vi "test.vi"() -> ()   [LabVIEW 2020]
panel:
  out "Array":i32[][](array[numeric])
  out "transposed array":i32[][](array[numeric])
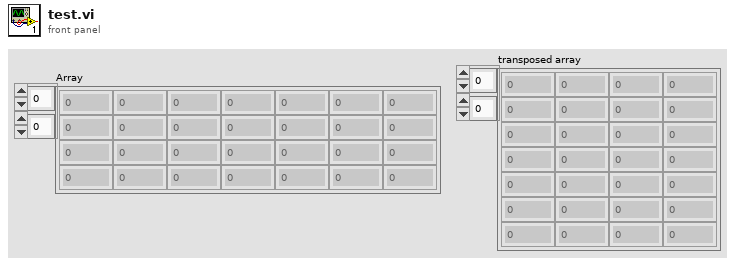
[diagram p1: front panel]
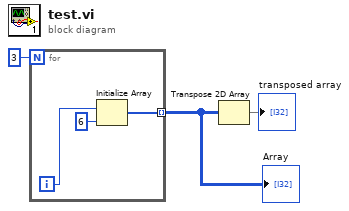
[diagram p0: block diagram]
diagram:
  n1 = for {
    N: 3 -> [_]
    tunnel: [w4] -> w2 mode=indexing
    i -> [w5]
    n2 = Initialize Array(w5, 6 ("dimension size")) -> (w4:i32[])
  }
  "Array" <- w2
  n3 = Transpose 2D Array(2D array=w2) -> (transposed array=→"transposed array":i32[][])
